vi "Filter by ADC Bounds.vi"(8 "error in (no error)":errorcluster, 9 "Min":u16, 10 "Max":u16, 11 "Entries":T1[](array[typedef])) -> (0 "error out":errorcluster, 3 "Filtered Entries":T1[](array[typedef]))   [LabVIEW 2019, in "Muon Data Post-Processing.lvlib"]
uses:
  File Entry.ctl
  Muon Data Post-Processing.lvlib
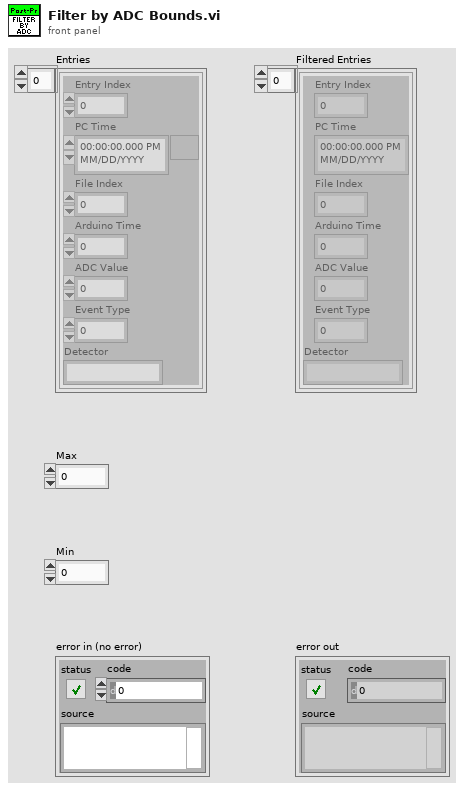
[diagram p1: front panel]
types:
  T1 = typedef "Muon Data Post-Processing.lvlib/File Entry.ctl" = cluster{"Entry Index":i32, "PC Time":timestamp, "File Index":i32, "Arduino Time":i32, "ADC Value":i32, "Event Type":i32, "Detector":string}
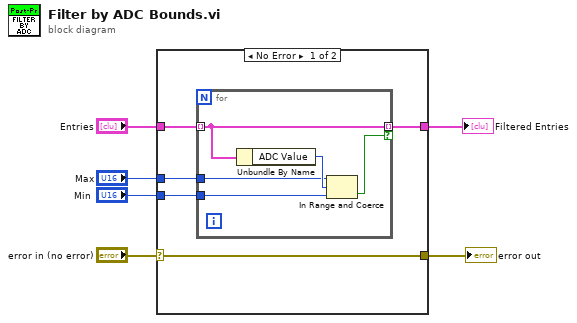
[diagram p0: block diagram]
diagram:
  n1 = case shown="No Error" "error in (no error)" {
    selector: "error in (no error)" -> [w11 w17]
    tunnel: [w11 w17] -> w5
    tunnel: "Entries" -> [w10 _]
    tunnel: "Max" -> [w9 _]
    tunnel: "Min" -> [w8 _]
    tunnel: [w7 _] -> w1
    frame No Error {
      n2 = for {
        tunnel: w10 -> [w16] mode=indexing
        tunnel: [w16] -> w7 mode=indexing if=w12
        tunnel: w9 -> [w14]
        tunnel: w8 -> [w13]
        n3 = Unbundle By Name(w16) -> ("ADC Value"=w15:i32)
        n4 = In Range and Coerce(upper limit=w14, x=w15, lower limit=w13) -> (In Range?=w12:bool)  [unwired: 1 out]
      }
    }
    frame Error {
    }
  }
  "error out" <- w5
  "Filtered Entries" <- w1
